vi "LambdaTemp2IR.vi"(8 "error constant":errorcluster, 9 "par 3":T1={"Loop time"={"Period [ms]"=5, "Processor"=-2}, "COM"={"COM IP"="192.168.8.70", "COM port"=30005, "Local port"=5556, "Next_IP 1"=0, "Next_IP 2"=0, "Next_IP 3"=0, "Next_IP 4"=0}, "O2Sensor1"={"Lambda"={"LSU4.2 Lambda"=[], "LSU4.2 Ip"=[], "LSU4.9 Lambda"=[], "LSU4.9 Ip"=[], "LZA03 Lambda"=[], "LZA03 Ip"=[], "LZA08 Lambda"=[], "LZA08 Ip"=[], "Custom Lambda"=[], "Custom Ip"=[]}, "Temp"={"LSU4.2 Temp"=[], "LSU4.2 Ohm"=[], "LSU4.9 Temp"=[], "LSU4.9 Ohm"=[], "LZA03 Temp"=[], "LZA03 Ohm"=[], "LZA08 Temp"=[], "LZA08 Ohm"=[], "Custom Temp"=[], "Custom Ohm"=[]}, "Lambda Type"=0, "PID"={"Ki"=0.0, "Kp"=0.0, "Kd"=0.0, "FeedFW"=0.0}}, "O2Sensor2"={"Lambda"={"LSU4.2 Lambda"=[], "LSU4.2 Ip"=[], "LSU4.9 Lambda"=[], "LSU4.9 Ip"=[], "LZA03 Lambda"=[], "LZA03 Ip"=[], "LZA08 Lambda"=[], "LZA08 Ip"=[], "Custom Lambda"=[], "Custom Ip"=[]}, "Temp"={"LSU4.2 Temp"=[], "LSU4.2 Ohm"=[], "LSU4.9 Temp"=[], "LSU4.9 Ohm"=[], "LZA03 Temp"=[], "LZA03 Ohm"=[], "LZA08 Temp"=[], "LZA08 Ohm"=[], "Custom Temp"=[], "Custom Ohm"=[]}, "Lambda Type"=0, "PID"={"Ki"=0.0, "Kp"=0.0, "Kd"=0.0, "FeedFW"=0.0}}, "O2Sensor3"={"Lambda"={"LSU4.2 Lambda"=[], "LSU4.2 Ip"=[], "LSU4.9 Lambda"=[], "LSU4.9 Ip"=[], "LZA03 Lambda"=[], "LZA03 Ip"=[], "LZA08 Lambda"=[], "LZA08 Ip"=[], "Custom Lambda"=[], "Custom Ip"=[]}, "Temp"={"LSU4.2 Temp"=[], "LSU4.2 Ohm"=[], "LSU4.9 Temp"=[], "LSU4.9 Ohm"=[], "LZA03 Temp"=[], "LZA03 Ohm"=[], "LZA08 Temp"=[], "LZA08 Ohm"=[], "Custom Temp"=[], "Custom Ohm"=[]}, "Lambda Type"=0, "PID"={"Ki"=0.0, "Kp"=0.0, "Kd"=0.0, "FeedFW"=0.0}}, "O2Sensor4"={"Lambda"={"LSU4.2 Lambda"=[], "LSU4.2 Ip"=[], "LSU4.9 Lambda"=[], "LSU4.9 Ip"=[], "LZA03 Lambda"=[], "LZA03 Ip"=[], "LZA08 Lambda"=[], "LZA08 Ip"=[], "Custom Lambda"=[], "Custom Ip"=[]}, "Temp"={"LSU4.2 Temp"=[], "LSU4.2 Ohm"=[], "LSU4.9 Temp"=[], "LSU4.9 Ohm"=[], "LZA03 Temp"=[], "LZA03 Ohm"=[], "LZA08 Temp"=[], "LZA08 Ohm"=[], "Custom Temp"=[], "Custom Ohm"=[]}, "Lambda Type"=0, "PID"={"Ki"=0.0, "Kp"=0.0, "Kd"=0.0, "FeedFW"=0.0}}, "Board"=0, "Mode"=enum."SLSC Mode", "vendor.Num"=4141, "product.Num"=0} {"Board" items=["O2Sim_2ch", "O2Sim_4ch"]; "O2Sensor4"."Lambda Type" items=["LSU4.2", "LSU4.9", "LZA03", "LZA08", "Custom", "[mA]"]; "O2Sensor3"."Lambda Type" items=["LSU4.2", "LSU4.9", "LZA03", "LZA08", "Custom", "[mA]"]; "O2Sensor2"."Lambda Type" items=["LSU4.2", "LSU4.9", "LZA03", "LZA08", "Custom", "[mA]"]; "O2Sensor1"."Lambda Type" items=["LSU4.2", "LSU4.9", "LZA03", "LZA08", "Custom", "[mA]"]}, 10 "SensorUsed":T3, 11 "VS control":dbl[](array[numeric])) -> (0 "error constant out":errorcluster, 3 "VS control out":dbl[](array[numeric]))   [LabVIEW 2017, in "ALMA_10201-10401_O2SensorSim Engine.lvlib"]
uses:
  ALMA_10201-10401_O2SensorSim Engine.lvlib
  Sensor_used.ctl
  Par.ctl
  LambdaType.ctl
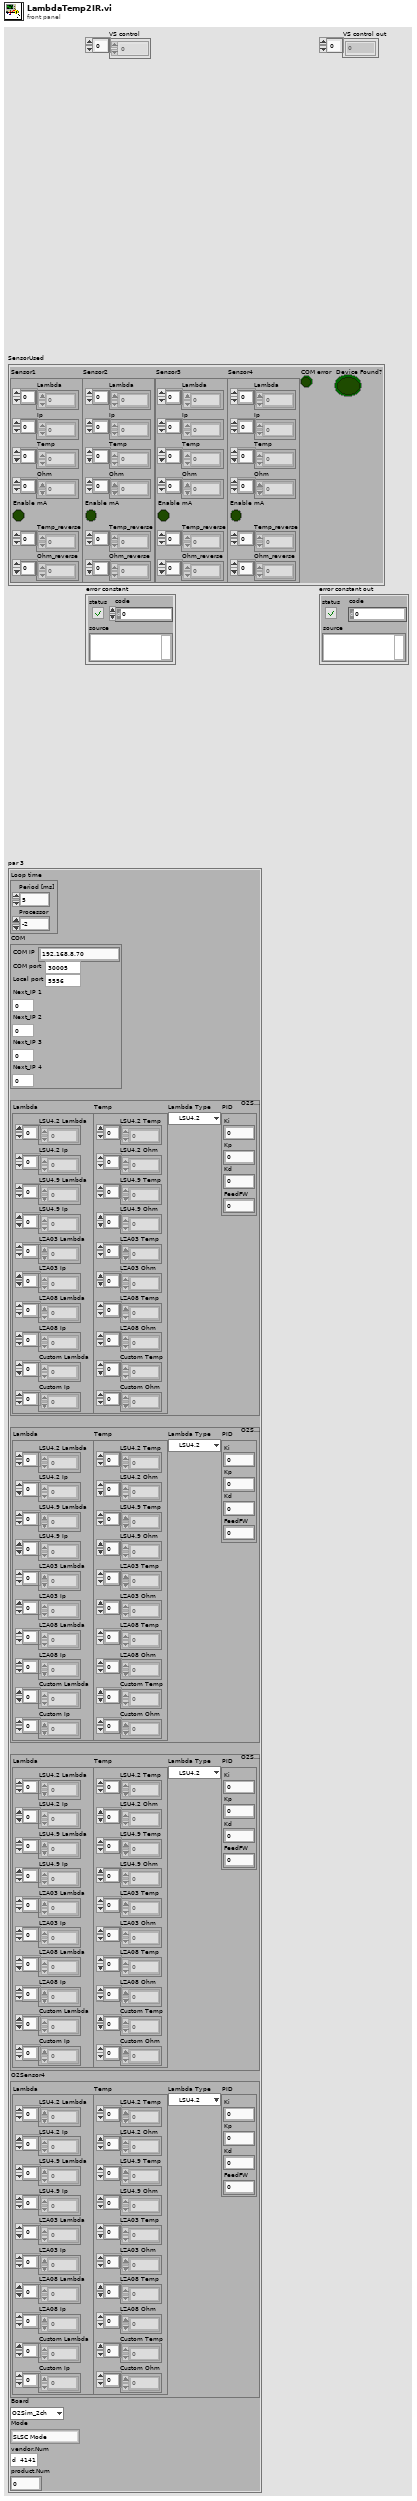
[diagram p1: front panel]
types:
  T1 = typedef "Par.ctl" = cluster{"Loop time":cluster{"Period [ms]":i64, "Processor":i32}, "COM":cluster{"COM IP":string, "COM port":u64, "Local port":u64, "Next_IP 1":u32, "Next_IP 2":u32, "Next_IP 3":u32, "Next_IP 4":u32}, "O2Sensor1":cluster{"Lambda":cluster{"LSU4.2 Lambda":dbl[], "LSU4.2 Ip":dbl[], "LSU4.9 Lambda":dbl[], "LSU4.9 Ip":dbl[], "LZA03 Lambda":dbl[], "LZA03 Ip":dbl[], "LZA08 Lambda":dbl[], "LZA08 Ip":dbl[], "Custom Lambda":dbl[], "Custom Ip":dbl[]}, "Temp":cluster{"LSU4.2 Temp":dbl[], "LSU4.2 Ohm":dbl[], "LSU4.9 Temp":dbl[], "LSU4.9 Ohm":dbl[], "LZA03 Temp":dbl[], "LZA03 Ohm":dbl[], "LZA08 Temp":dbl[], "LZA08 Ohm":dbl[], "Custom Temp":dbl[], "Custom Ohm":dbl[]}, "Lambda Type":T2, "PID":cluster{"Ki":dbl, "Kp":dbl, "Kd":dbl, "FeedFW":dbl}}, "O2Sensor2":cluster{"Lambda":cluster{"LSU4.2 Lambda":dbl[], "LSU4.2 Ip":dbl[], "LSU4.9 Lambda":dbl[], "LSU4.9 Ip":dbl[], "LZA03 Lambda":dbl[], "LZA03 Ip":dbl[], "LZA08 Lambda":dbl[], "LZA08 Ip":dbl[], "Custom Lambda":dbl[], "Custom Ip":dbl[]}, "Temp":cluster{"LSU4.2 Temp":dbl[], "LSU4.2 Ohm":dbl[], "LSU4.9 Temp":dbl[], "LSU4.9 Ohm":dbl[], "LZA03 Temp":dbl[], "LZA03 Ohm":dbl[], "LZA08 Temp":dbl[], "LZA08 Ohm":dbl[], "Custom Temp":dbl[], "Custom Ohm":dbl[]}, "Lambda Type":T2, "PID":cluster{"Ki":dbl, "Kp":dbl, "Kd":dbl, "FeedFW":dbl}}, "O2Sensor3":cluster{"Lambda":cluster{"LSU4.2 Lambda":dbl[], "LSU4.2 Ip":dbl[], "LSU4.9 Lambda":dbl[], "LSU4.9 Ip":dbl[], "LZA03 Lambda":dbl[], "LZA03 Ip":dbl[], "LZA08 Lambda":dbl[], "LZA08 Ip":dbl[], "Custom Lambda":dbl[], "Custom Ip":dbl[]}, "Temp":cluster{"LSU4.2 Temp":dbl[], "LSU4.2 Ohm":dbl[], "LSU4.9 Temp":dbl[], "LSU4.9 Ohm":dbl[], "LZA03 Temp":dbl[], "LZA03 Ohm":dbl[], "LZA08 Temp":dbl[], "LZA08 Ohm":dbl[], "Custom Temp":dbl[], "Custom Ohm":dbl[]}, "Lambda Type":T2, "PID":cluster{"Ki":dbl, "Kp":dbl, "Kd":dbl, "FeedFW":dbl}}, "O2Sensor4":cluster{"Lambda":cluster{"LSU4.2 Lambda":dbl[], "LSU4.2 Ip":dbl[], "LSU4.9 Lambda":dbl[], "LSU4.9 Ip":dbl[], "LZA03 Lambda":dbl[], "LZA03 Ip":dbl[], "LZA08 Lambda":dbl[], "LZA08 Ip":dbl[], "Custom Lambda":dbl[], "Custom Ip":dbl[]}, "Temp":cluster{"LSU4.2 Temp":dbl[], "LSU4.2 Ohm":dbl[], "LSU4.9 Temp":dbl[], "LSU4.9 Ohm":dbl[], "LZA03 Temp":dbl[], "LZA03 Ohm":dbl[], "LZA08 Temp":dbl[], "LZA08 Ohm":dbl[], "Custom Temp":dbl[], "Custom Ohm":dbl[]}, "Lambda Type":T2, "PID":cluster{"Ki":dbl, "Kp":dbl, "Kd":dbl, "FeedFW":dbl}}, "Board":u16, "Mode":enum16{"SLSC Mode", "ANALOG Mode"}, "vendor.Num":u32, "product.Num":u32}
  T2 = typedef "LambdaType.ctl" = u16
  T3 = typedef "ALMA_10201-10401_O2SensorSim Engine.lvlib/Sensor_used.ctl" = cluster{"Sensor1":cluster{"Lambda":dbl[], "Ip":dbl[], "Temp":dbl[], "Ohm":dbl[], "Enable mA":bool, "Temp_reverse":dbl[], "Ohm_reverse":dbl[]}, "Sensor2":cluster{"Lambda":dbl[], "Ip":dbl[], "Temp":dbl[], "Ohm":dbl[], "Enable mA":bool, "Temp_reverse":dbl[], "Ohm_reverse":dbl[]}, "Sensor3":cluster{"Lambda":dbl[], "Ip":dbl[], "Temp":dbl[], "Ohm":dbl[], "Enable mA":bool, "Temp_reverse":dbl[], "Ohm_reverse":dbl[]}, "Sensor4":cluster{"Lambda":dbl[], "Ip":dbl[], "Temp":dbl[], "Ohm":dbl[], "Enable mA":bool, "Temp_reverse":dbl[], "Ohm_reverse":dbl[]}, "COM error":bool, "Device Found?":bool}
  T4 = cluster{"Lambda":dbl[], "Ip":dbl[], "Temp":dbl[], "Ohm":dbl[], "Enable mA":bool, "Temp_reverse":dbl[], "Ohm_reverse":dbl[]}
  T5 = cluster{"Lambda":dbl[], "Ip":dbl[], "Temp":dbl[], "Ohm":dbl[], "Enable mA":bool, "Temp_reverse":dbl[], "Ohm_reverse":dbl[]}[]
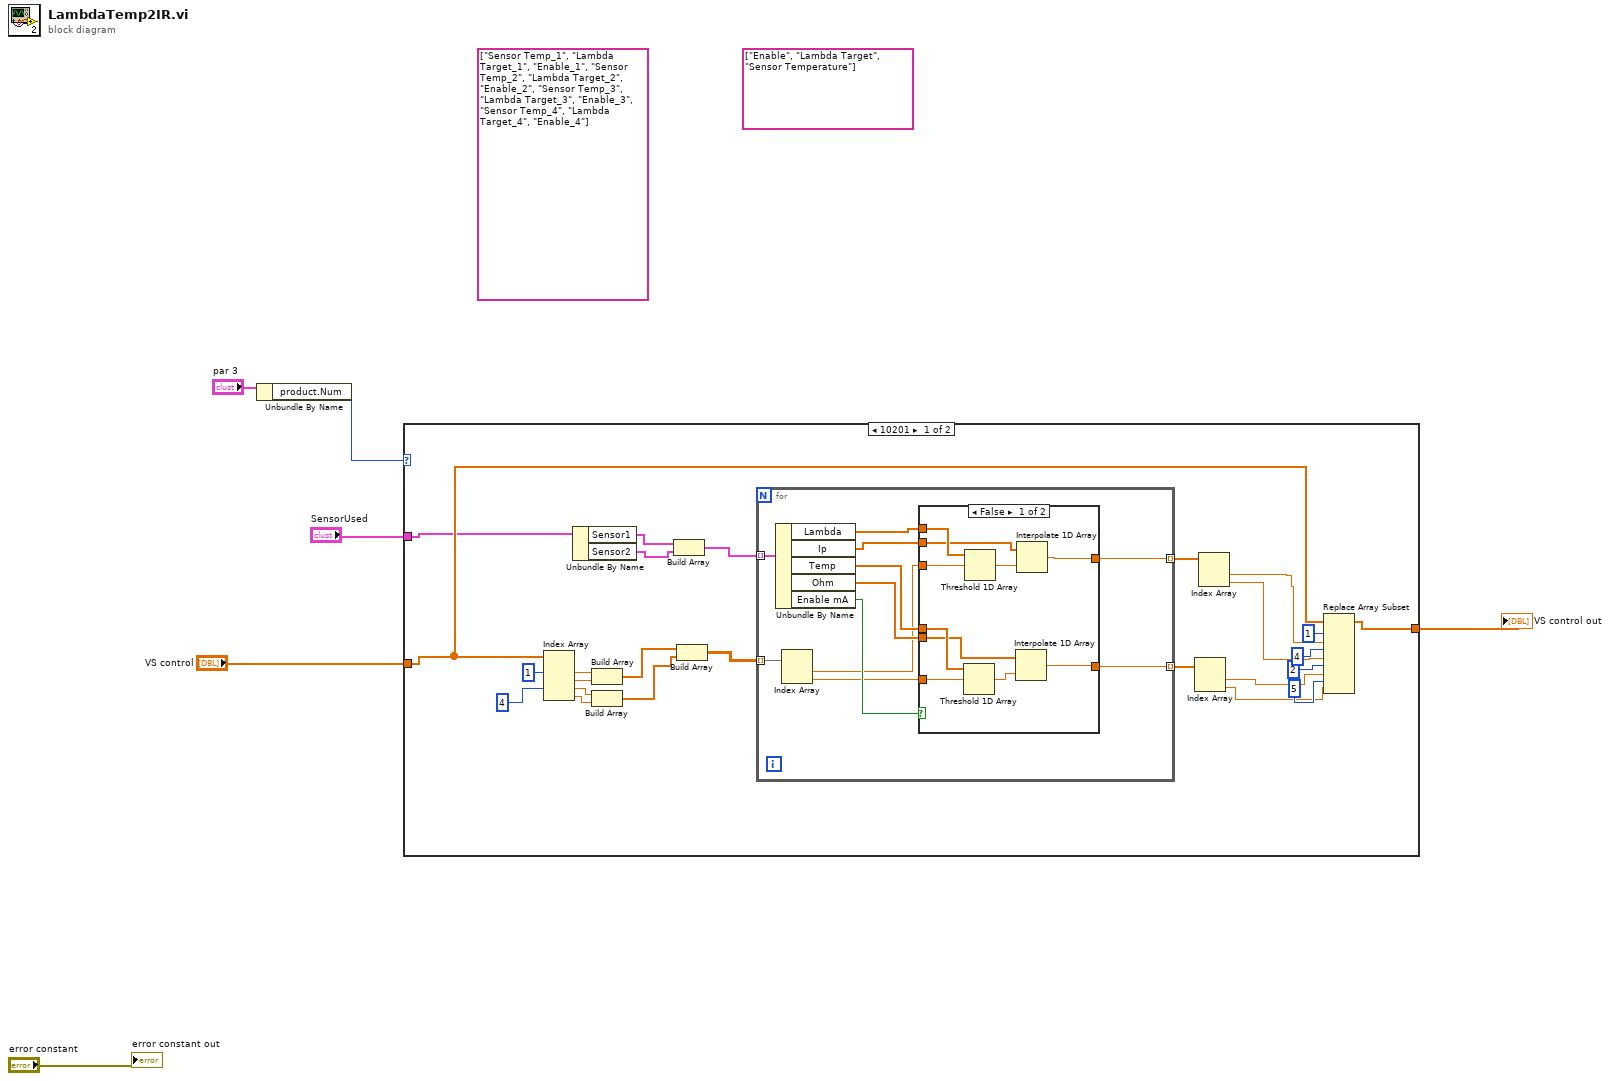
[diagram p0: block diagram]
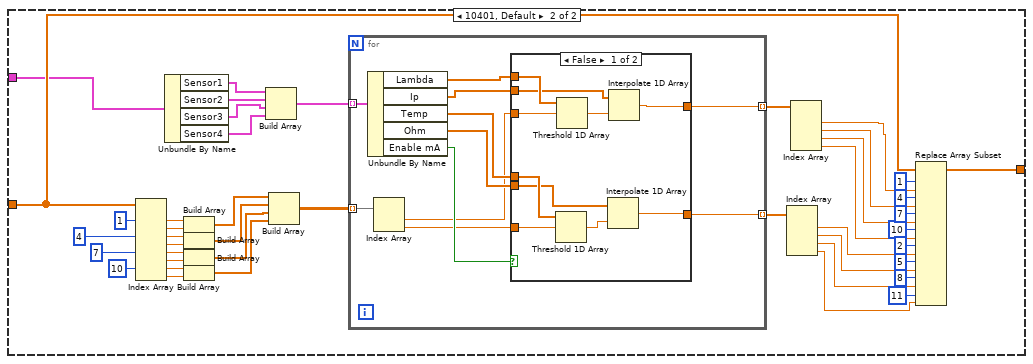
[diagram p3: hidden frame]
diagram:
  (unwired) string[] ["Enable", "Lambda Target", "Sensor Temperature"] ("O2SensoSim Setpoint 2")
  (unwired) string[] ["Sensor Temp_1", "Lambda Target_1", "Enable_1", "Sensor Temp_2", "Lambda Target_2", "Enable_2", "Sensor Temp_3", "Lambda Target_3", "Enable_3", "Sensor Temp_4", "Lambda Target_4", "Enable_4"] ("O2SensoSim Setpoint 2")
  n1 = Unbundle By Name("par 3") -> ("product.Num"=w2:u32)
  n2 = case shown="10201" w2 {
    tunnel: "VS control" -> [w11 w75]
    tunnel: [w10 w72] -> w5
    tunnel: "SensorUsed" -> [w7 w55]
    frame 10201 {
      n3 = Index Array(array=w11, index #1=1 ("index"), index #3=4 ("index")) -> (element #1=w24:dbl, element #2=w23:dbl, element #3=w29:dbl, element #4=w30:dbl)  [unwired: 2 in]
      n4 = Unbundle By Name(w7) -> ("Sensor1"=w28:T4, "Sensor2"=w27:T4)
      n5 = Build Array(w24, w23) -> (w25:dbl[])
      n6 = Build Array(w29, w30) -> (w22:dbl[])
      n7 = Build Array(w28, w27) -> (w26:T5)
      n8 = Build Array(w25, w22) -> (w21:dbl[][])
      n9 = for {
        tunnel: w26 -> [w42] mode=indexing
        tunnel: w21 -> [w40] mode=indexing
        tunnel: [w33] -> w20 mode=indexing
        tunnel: [w32] -> w19 mode=indexing
        n10 = Unbundle By Name(w42) -> ("Lambda"=w39:dbl[], "Ip"=w38:dbl[], "Temp"=w37:dbl[], "Ohm"=w36:dbl[], "Enable mA"=w41:bool)
        n11 = Index Array(array=w40) -> (element #1=w35:dbl, element #2=w34:dbl)  [unwired: 2 in]
        n12 = case shown="False" w41 {
          tunnel: w35 -> [w51 w54]
          tunnel: w34 -> [w49 w53]
          tunnel: [w48 w54] -> w33
          tunnel: [w47 w53] -> w32
          tunnel: w39 -> [w46 _]
          tunnel: w38 -> [w45 _]
          tunnel: w37 -> [w44 _]
          tunnel: w36 -> [w43 _]
          frame False {
            n13 = Threshold 1D Array(2:w49, 3:w44) -> (0:w50:dbl)  [unwired: 1 in]
            n14 = Threshold 1D Array(2:w51, 3:w46) -> (0:w52:dbl)  [unwired: 1 in]
            n15 = Interpolate 1D Array(1:w50, 2:w43) -> (0:w47:dbl)
            n16 = Interpolate 1D Array(1:w52, 2:w45) -> (0:w48:dbl)
          }
          frame True {
          }
        }
      }
      n17 = Index Array(array=w19) -> (element #1=w31:dbl, element #2=w8:dbl)  [unwired: 2 in]
      n18 = Index Array(array=w20) -> (element #1=w18:dbl, element #2=w9:dbl)  [unwired: 2 in]
      n19 = Replace Array Subset(array=w11, new element #1=w18, index #1=1 ("index"), new element #2=w9, index #2=4 ("index"), new element #3=w31, index #3=2 ("index"), new element #4=w8, index #4=5 ("index")) -> (w10:dbl[])
    }
    frame 10401, Default {
      n20 = Index Array(array=w75, index #1=1 ("index"), index #3=4 ("index"), index #5=7 ("index"), index #7=10 ("index")) -> (element #1=w87:dbl, element #2=w86:dbl, element #3=w85:dbl, element #4=w84:dbl, element #5=w83:dbl, element #6=w82:dbl, element #7=w81:dbl, element #8=w80:dbl)  [unwired: 4 in]
      n21 = Unbundle By Name(w55) -> ("Sensor1"=w97:T4, "Sensor2"=w96:T4, "Sensor3"=w95:T4, "Sensor4"=w94:T4)
      n22 = Build Array(w87, w86) -> (w92:dbl[])
      n23 = Build Array(w85, w84) -> (w79:dbl[])
      n24 = Build Array(w83, w82) -> (w78:dbl[])
      n25 = Build Array(w81, w80) -> (w77:dbl[])
      n26 = Build Array(w97, w96, w95, w94) -> (w93:T5)
      n27 = Build Array(w92, w79, w78, w77) -> (w76:dbl[][])
      n28 = for {
        tunnel: w93 -> [w108] mode=indexing
        tunnel: w76 -> [w106] mode=indexing
        tunnel: [w99] -> w74 mode=indexing
        tunnel: [w98] -> w73 mode=indexing
        n29 = Unbundle By Name(w108) -> ("Lambda"=w105:dbl[], "Ip"=w104:dbl[], "Temp"=w103:dbl[], "Ohm"=w102:dbl[], "Enable mA"=w107:bool)
        n30 = Index Array(array=w106) -> (element #1=w101:dbl, element #2=w100:dbl)  [unwired: 2 in]
        n31 = case shown="False" w107 {
          tunnel: w101 -> [w117 w120]
          tunnel: w100 -> [w115 w119]
          tunnel: [w114 w120] -> w99
          tunnel: [w113 w119] -> w98
          tunnel: w105 -> [w112 _]
          tunnel: w104 -> [w111 _]
          tunnel: w103 -> [w110 _]
          tunnel: w102 -> [w109 _]
          frame False {
            n32 = Threshold 1D Array(2:w115, 3:w110) -> (0:w116:dbl)  [unwired: 1 in]
            n33 = Threshold 1D Array(2:w117, 3:w112) -> (0:w118:dbl)  [unwired: 1 in]
            n34 = Interpolate 1D Array(1:w116, 2:w109) -> (0:w113:dbl)
            n35 = Interpolate 1D Array(1:w118, 2:w111) -> (0:w114:dbl)
          }
          frame True {
          }
        }
      }
      n36 = Index Array(array=w73) -> (element #1=w59:dbl, element #2=w58:dbl, element #3=w57:dbl, element #4=w56:dbl)  [unwired: 4 in]
      n37 = Index Array(array=w74) -> (element #1=w63:dbl, element #2=w62:dbl, element #3=w61:dbl, element #4=w60:dbl)  [unwired: 4 in]
      n38 = Replace Array Subset(array=w75, new element #1=w63, index #1=1 ("index"), new element #2=w62, index #2=4 ("index"), new element #3=w61, index #3=7 ("index"), new element #4=w60, index #4=10 ("index"), new element #5=w59, index #5=2 ("index"), new element #6=w58, index #6=5 ("index"), new element #7=w57, index #7=8 ("index"), new element #8=w56, index #8=11 ("index")) -> (w72:dbl[])
    }
  }
  "VS control out" <- w5
  "error constant out" <- "error constant"
